vi "Measure Voltage.vi"(8 "error in (no error)":errorcluster, 11 "Low Level PSU In":refnum<class "Low Level PSU.lvclass">) -> (0 "error out":errorcluster, 2 "Output Voltage":dbl format="%.4f", 3 "Low Level PSU Out":refnum<class "Low Level PSU.lvclass">)   [LabVIEW 2020, in "Low Level PSU With Tests.lvlib" / "Low Level PSU.lvclass"]
uses:
  Low Level PSU.lvclass
  Low Level PSU.lvclass/Low Level PSU.ctl
  Instrument Interface/Instrument Interface.lvclass
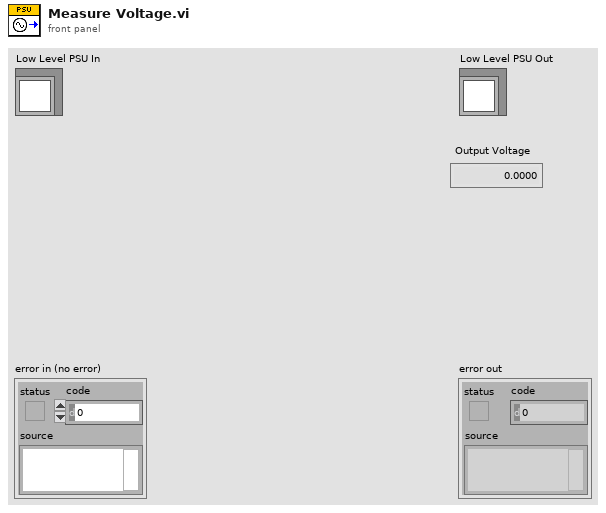
[diagram p1: front panel]
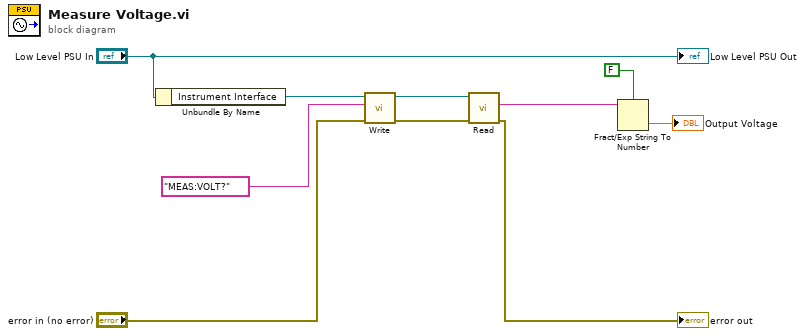
[diagram p0: block diagram]
diagram:
  n1 = Unbundle By Name("Low Level PSU In") -> ("Instrument Interface"=w5:refnum<class "Instrument Interface.lvclass">)
  n2 = call-dynamic "Write.vi"("error in (no error)"="error in (no error)", "Data"="MEAS:VOLT?" ("format string"), "Instrument Interface in"=w5) -> ("error out"=w9:errorcluster, "Instrument Interface out"=w10:refnum<class "Instrument Interface.lvclass">)  [unwired: 7 in]
  n3 = call-dynamic "Read.vi"("error in (no error)"=w9, "Instrument Interface in"=w10) -> ("error out"=→"error out":errorcluster, "Data"=w1:string)  [unwired: 7 in, 1 out]
  n4 = Fract/Exp String To Number(use system decimal point (T)=FALSE, string=w1) -> (number=→"Output Voltage":dbl)  [unwired: 2 in, 1 out]
  "Low Level PSU Out" <- "Low Level PSU In"
